vi "isPathExist.vi"(3 "Array":path[](array[path])) -> (1 "Numeric":i16)   [LabVIEW 2014]
doc: "André Romero - 2017\nandretec@ifsc.usp.br"
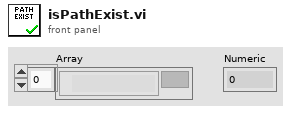
[diagram p1: front panel]
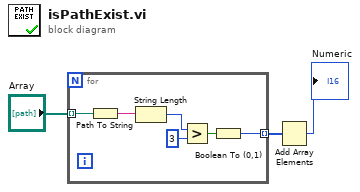
[diagram p0: block diagram]
diagram:
  n1 = for {
    tunnel: "Array" -> [w6] mode=indexing
    tunnel: [w4] -> w1 mode=indexing
    n2 = Path To String(path=w6) -> (string=w9:string)
    n3 = String Length(string=w9) -> (length=w8:i32)
    n4 = Greater?(x=w8, y=3) -> (0:w5:bool)
    n5 = Boolean To (0,1)(Boolean=w5) -> (0, 1=w4:i16)
  }
  n6 = Add Array Elements(numeric array=w1) -> (sum=→"Numeric":i16)
